vi "Fz_Zeichnen.vi"(11 "Lenkwinkel [rad]":dbl) -> (1 "Breite Sensor/2 [cm] out":dbl=6.0, 2 "Achsabstand [cm] out":dbl=22.0, 3 "Fz":dbl[][][](array[numeric]))   [LabVIEW 2019]
uses:
  <vilib>/Analysis/baseanly.llb/Real A x B.vi
  <vilib>/Analysis/Matrix/Numeric/Add/Add - RM,RM.vi
  <vilib>/Analysis/NI_AALBase.lvlib
  <vilib>/Analysis/Matrix/NI_Matrix.lvlib
panel:
  out "XY Graph":cluster{"x":dbl[], "y":dbl[]}[](graph)
  in  "Breite Sensor/2 [cm]":dbl=6.0
  in  "Sensorabstand von Hinterachse":dbl=23.0
  in  "Radbreite":dbl=1.0
  in  "Radradius":dbl=3.0
  in  "Achsabstand [cm]":dbl=22.0
  in  "Spurbreite/2 [cm]":dbl=8.0
  # "alles in cm"
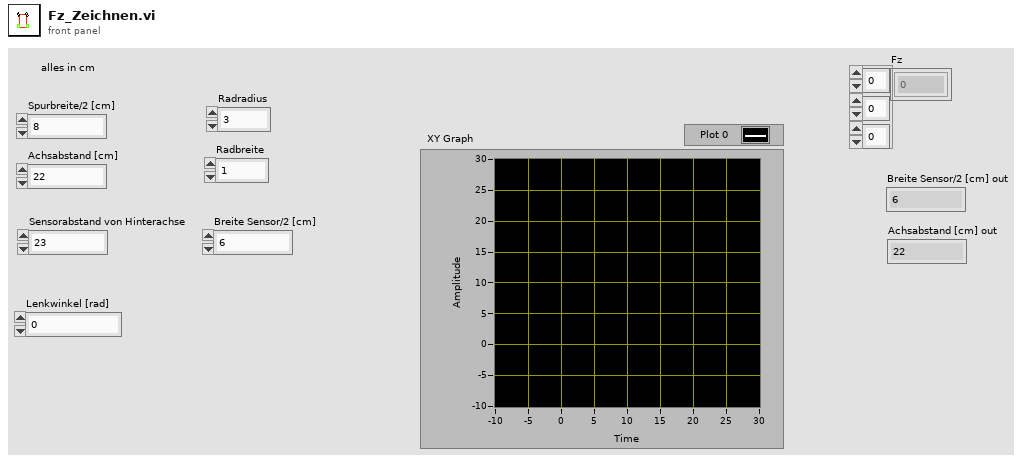
[diagram p1: front panel]
types:
  T1 = typedef "NI_Matrix.lvlib/RealMatrix.ctl" = dbl[][]
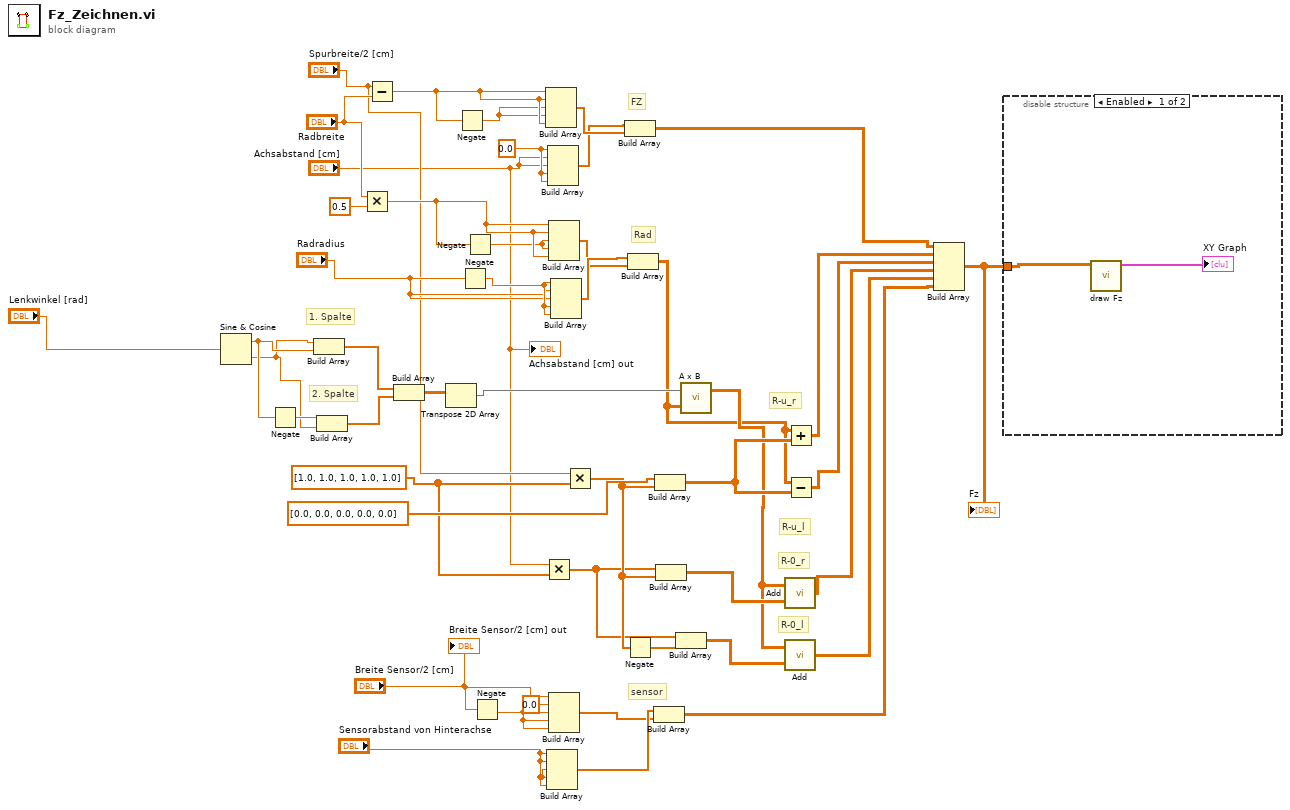
[diagram p0: block diagram]
diagram:
  w22 = dbl[] [1.0, 1.0, 1.0, 1.0, 1.0]
  w44 = 0.0
  # "R-0_l"
  # "R-0_r"
  # "R-u_l"
  # "R-u_r"
  # "2. Spalte"
  # "1. Spalte"
  # "sensor"
  # "Rad"
  # "FZ"
  n1 = Sine & Cosine(0:"Lenkwinkel [rad]") -> (1:w32:dbl, 2:w30:dbl)
  n2 = Negate(x=w32) -> (-x=w31:dbl)
  n3 = Build Array(w30, w32) -> (w29:dbl[])
  n4 = Build Array(w31, w30) -> (w28:dbl[])
  n5 = Multiply(x="Radbreite", y=0.5) -> (x*y=w37:dbl)
  n6 = Subtract(x="Spurbreite/2 [cm]", y="Radbreite") -> (x-y=w46:dbl)
  n7 = Build Array(w29, w28) -> (w27:dbl[][])
  n8 = Transpose 2D Array(2D array=w27) -> (transposed array=w26:dbl[][])
  n9 = Negate(x=w46) -> (-x=w45:dbl)
  n10 = Negate(x="Radradius") -> (-x=w35:dbl)
  n11 = Negate(x=w37) -> (-x=w36:dbl)
  n12 = Negate(x="Breite Sensor/2 [cm]") -> (-x=w2:dbl)
  n13 = Multiply(x="Achsabstand [cm]", y=w22) -> (x*y=w17:dbl[])
  n14 = Build Array(w46, w46, w45, w45, w46) -> (w43:dbl[])
  n15 = Build Array("Sensorabstand von Hinterachse", "Sensorabstand von Hinterachse", "Sensorabstand von Hinterachse", "Sensorabstand von Hinterachse", "Sensorabstand von Hinterachse") -> (w13:dbl[])
  n16 = Build Array(w44, "Achsabstand [cm]", "Achsabstand [cm]", w44, w44) -> (w42:dbl[])
  n17 = Build Array(w37, w37, w36, w36, w37) -> (w40:dbl[])
  n18 = Build Array("Breite Sensor/2 [cm]", 0.0 ("element"), w2, w2, w2) -> (w12:dbl[])
  n19 = Build Array(w35, "Radradius", "Radradius", w35, w35) -> (w41:dbl[])
  n20 = Multiply(x="Spurbreite/2 [cm]", y=w22) -> (x*y=w19:dbl[])
  n21 = Build Array(w42, w43) -> (w11:dbl[][])
  n22 = Negate(x=w19) -> (-x=w18:dbl[])
  n23 = Build Array(w41, w40) -> (w4:dbl[][])
  n24 = Build Array(w13, w12) -> (w6:dbl[][])
  n25 = Build Array(dbl[] [0.0, 0.0, 0.0, 0.0, 0.0], w19) -> (w23:dbl[][])
  n26 = Build Array(w17, w19) -> (w20:dbl[][])
  n27 = Build Array(w17, w18) -> (w16:dbl[][])
  n28 = call-poly <vilib>:"A x B.vi"("B"=w4, "A"=w26) -> ("A x B"=w15:T1)  [unwired: 1 out]
  n29 = call-poly <vilib>:"Add.vi"("Real Matrix B"=w20, "Real Matrix A"=w15) -> ("A + B"=w8:T1)
  n30 = call-poly <vilib>:"Add.vi"("Real Matrix B"=w16, "Real Matrix A"=w15) -> ("A + B"=w7:T1)
  n31 = Add ("Add.vi")(x=w4, y=w23) -> (x+y=w10:dbl[][])
  n32 = Subtract ("Subtract.vi")(x=w4, y=w23) -> (x-y=w9:dbl[][])
  n33 = Build Array(w11, w10, w9, w8, w7, w6) -> (w5:dbl[][][])
  "Fz" <- w5
  n34 = disable-structure shown="Enabled" {
    disable-tunnel: w5 -> [w48 _]
    frame Enabled {
      n35 = call "draw Fz.vi"("FZ"=w48) -> ("X_Y_Plot"=→"XY Graph":cluster{"x":dbl[], "y":dbl[]}[])  [unwired: 10 in]
    }
    frame Disabled {
    }
  }
  "Breite Sensor/2 [cm] out" <- "Breite Sensor/2 [cm]"
  "Achsabstand [cm] out" <- "Achsabstand [cm]"
